vi "dIMU_Accel_Poly.vi"   [LabVIEW 2010]
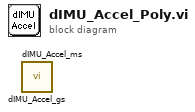
[diagram p0: block diagram]
diagram:
  n1 = call "dIMU_Accel_ms.vi"() -> ()  [unwired: 8 in, 4 out]
  n2 = call "dIMU_Accel_gs.vi"() -> ()  [unwired: 8 in, 4 out]
